vi "SplitFileStringProj1.vi"(0 "String from file":string) -> (9 "Voltage (X)":dbl[](array[numeric]), 11 "Current (Y)":dbl[](array[numeric]), 14 "Name":string, 15 "Part":string, 16 "Datum a cas mereni":string, 17 "Minimalni napeti":string, 18 "Maximalni napeti":string, 19 "Krok":string)   [LabVIEW 2021]
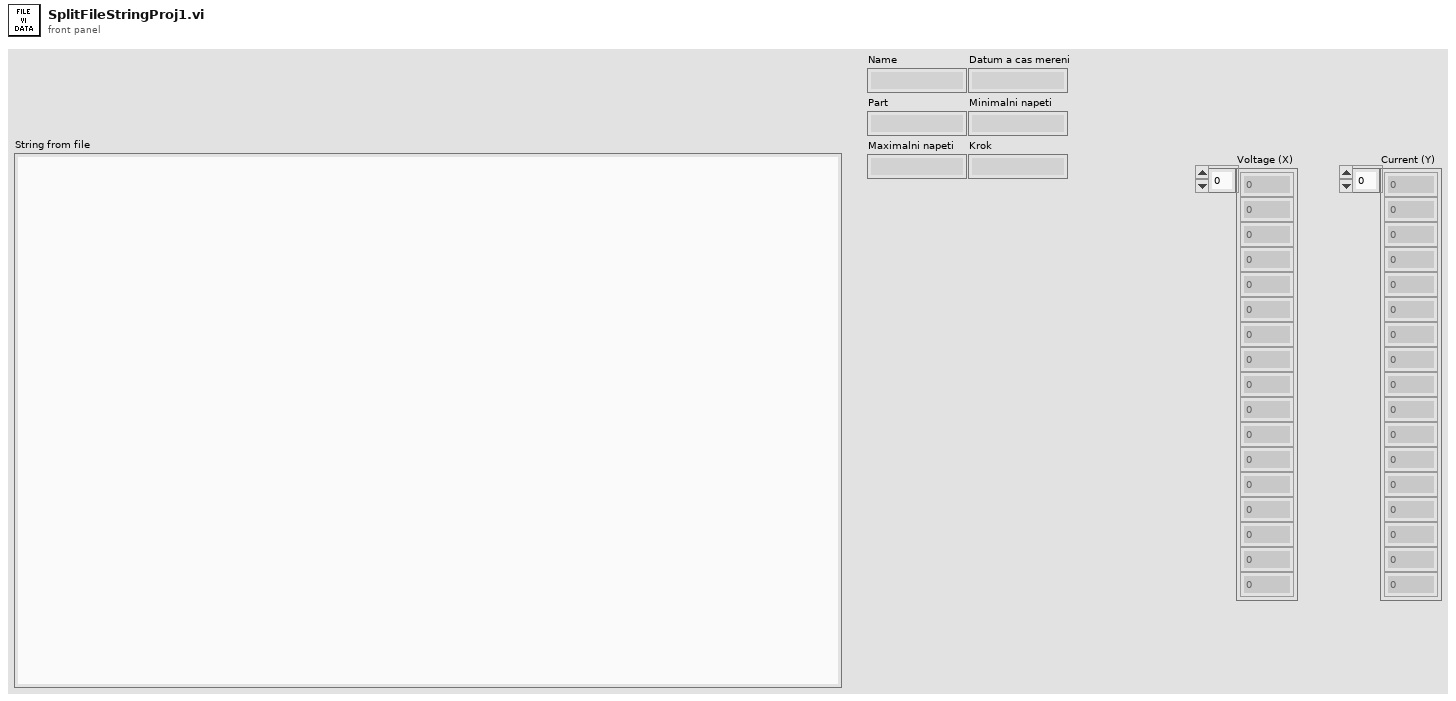
[diagram p1: front panel]
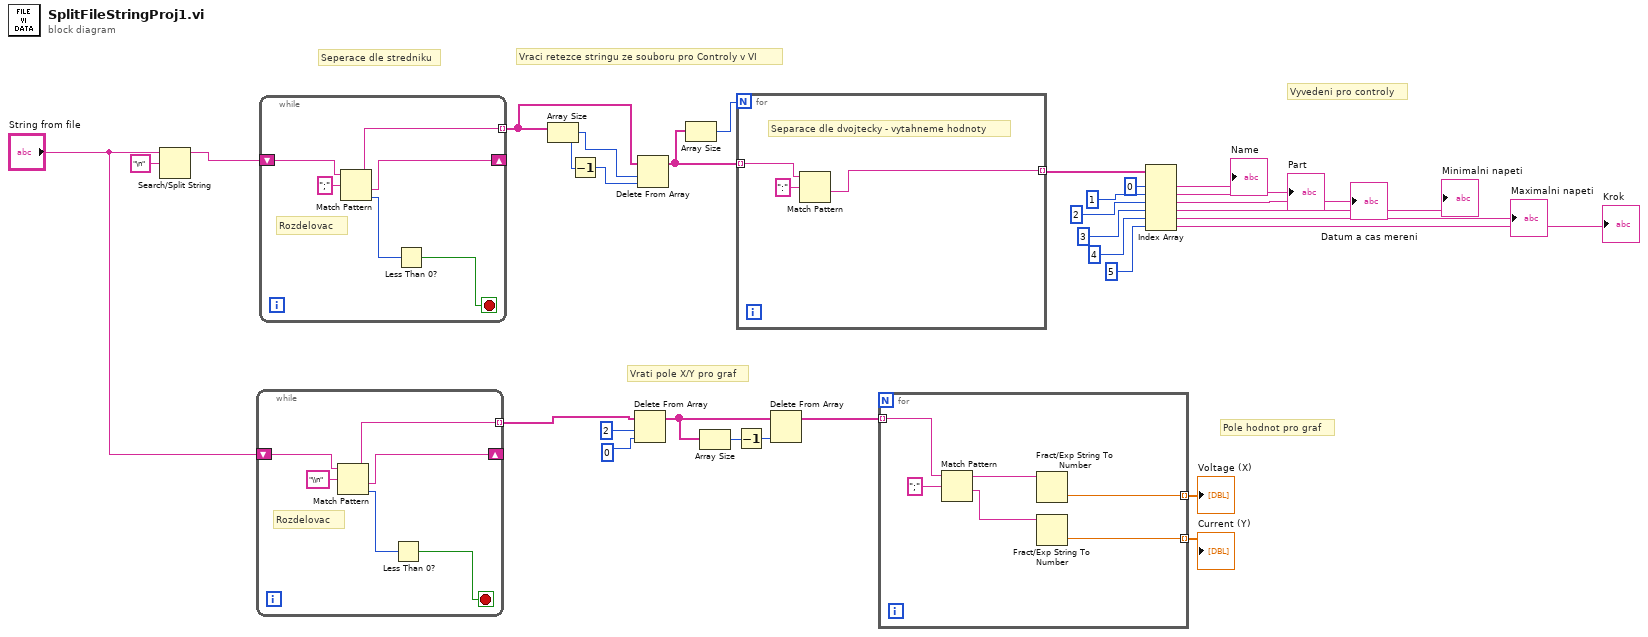
[diagram p0: block diagram]
diagram:
  # "Seperace dle stredniku"
  # "Pole hodnot pro graf"
  # "Vyvedeni pro controly"
  # "Vrati pole X/Y pro graf"
  # "Vraci retezce stringu ze souboru pro Controly v VI"
  n1 = Search/Split String(string="String from file", search string/char (-)="\n") -> (substring before match=w11:string)  [unwired: 1 in, 2 out]
  n2 = while {
    shift-right: [w32] -> _
    shift-left: "String from file" -> [w33]
    tunnel: [w31] -> w7 mode=indexing
    stop <- w34 stop-if-true
    # "Rozdelovac"
    n3 = Match Pattern(string=w33, regular expression="\\n") -> (before substring=w31:string, after substring=w32:string, offset past match=w35:i32)  [unwired: 1 in, 1 out]
    n4 = Less Than 0?(x=w35) -> (x < 0?=w34:bool)
  }
  n5 = while {
    shift-right: [w38] -> _
    shift-left: w11 -> [w39]
    tunnel: [w37] -> w28 mode=indexing
    stop <- w40 stop-if-true
    # "Rozdelovac"
    n6 = Match Pattern(string=w39, regular expression=";") -> (before substring=w37:string, after substring=w38:string, offset past match=w41:i32)  [unwired: 1 in, 1 out]
    n7 = Less Than 0?(x=w41) -> (x < 0?=w40:bool)
  }
  n8 = Array Size(array=w28) -> (size(s)=w27:i32)
  n9 = Decrement(x=w27) -> (x-1=w29:i32)
  n10 = Delete From Array(array=w7, length=2, index=0) -> (array with subset deleted=w4:string[])  [unwired: 1 out]
  n11 = Delete From Array(array=w28, length=w27, index=w29) -> (array with subset deleted=w25:string[])  [unwired: 1 out]
  n12 = Array Size(array=w25) -> (size(s)=w26:i32)
  n13 = Array Size(array=w4) -> (size(s)=w6:i32)
  n14 = Decrement(x=w6) -> (x-1=w5:i32)
  n15 = for {
    N: w26 -> [_]
    tunnel: w25 -> [w45] mode=indexing
    tunnel: [w43] -> w24 mode=indexing
    # "Separace dle dvojtecky - vytahneme hodnoty"
    n16 = Match Pattern(string=w45, regular expression=":") -> (after substring=w43:string)  [unwired: 1 in, 3 out]
  }
  n17 = Delete From Array(array=w4, index=w5) -> (array with subset deleted=w3:string[])  [unwired: 1 in, 1 out]
  n18 = for {
    tunnel: w3 -> [w50] mode=indexing
    tunnel: [w47] -> w2 mode=indexing
    tunnel: [w46] -> w1 mode=indexing
    n19 = Match Pattern(string=w50, regular expression=";") -> (before substring=w49:string, after substring=w48:string)  [unwired: 1 in, 2 out]
    n20 = Fract/Exp String To Number(string=w49) -> (number=w47:dbl)  [unwired: 3 in, 1 out]
    n21 = Fract/Exp String To Number(string=w48) -> (number=w46:dbl)  [unwired: 3 in, 1 out]
  }
  "Voltage (X)" <- w2
  "Current (Y)" <- w1
  n22 = Index Array(array=w24, index #1=0 ("index"), index #2=1 ("index"), index #3=2 ("index"), index #4=3 ("index"), index #5=4 ("index"), index #6=5 ("index")) -> (element #1=→"Name":string, element #2=→"Part":string, element #3=→"Datum a cas mereni":string, element #4=→"Minimalni napeti":string, element #5=→"Maximalni napeti":string, element #6=→"Krok":string)
